vi "CT-Sweep One Component (LUT).vi"(0 "Phase In":dbl=100000.0, 1 "factors":dbl[](array[numeric]), 5 "Last Freq (Hz)":dbl=100000.0, 7 "New Freq (Hz)":dbl=100000.0, 9 "dt (s)":dbl=100000.0, 11 "Npts":i32, 13 "randomize phase":bool) -> (4 "Phase Out":dbl, 8 "Y":dbl[](array[numeric]))   [LabVIEW 2015]
uses:
  CT-Globals.vi
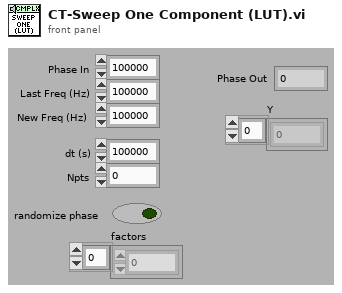
[diagram p1: front panel]
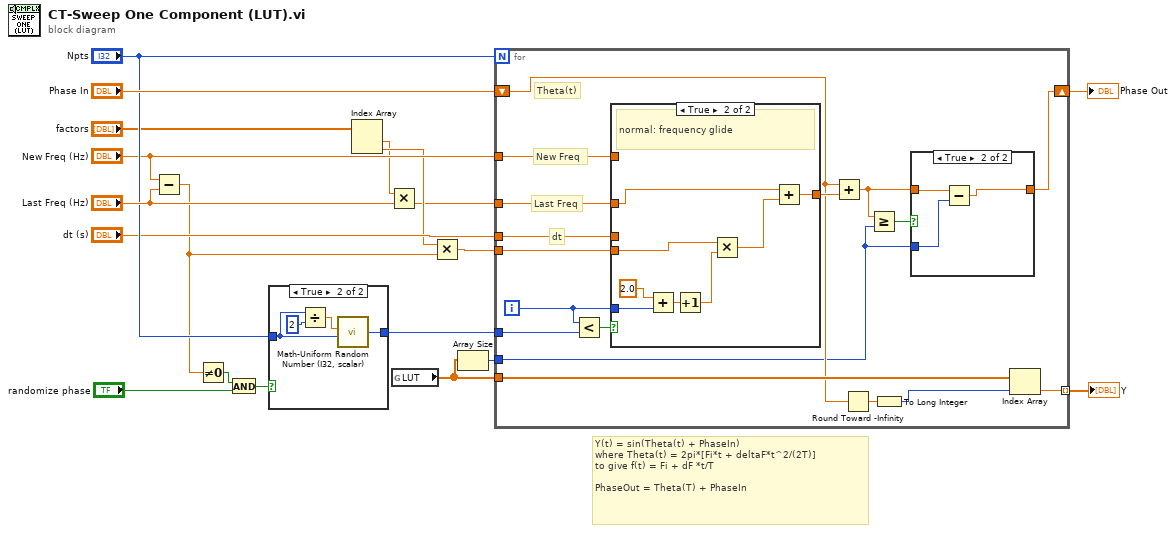
[diagram p0: block diagram]
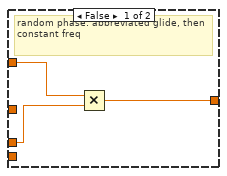
[diagram p4: hidden frame]
diagram:
  # "Y(t) = sin(Theta(t) + PhaseIn)\nwhere Theta(t) = 2pi*[Fi*t + deltaF*t^2/(2T)]\nto give f(t) = Fi + dF *t/T \n\nPhaseOut = Theta(T) + PhaseIn"
  n1 = Subtract(x="New Freq (Hz)", y="Last Freq (Hz)") -> (x-y=w4:dbl)
  n2 = Not Equal To 0?(x=w4) -> (x != 0?=w12:bool)
  n3 = And(x=w12, y="randomize phase") -> (x .and. y?=w13:bool)
  n4 = case shown="True" w13 {
    tunnel: "Npts" -> [w20 w23]
    tunnel: [w20 w21] -> w14
    frame False {
    }
    frame True {
      n5 = Divide(x=w23, y=2) -> (x/y=w22:dbl)
      n6 = call "Math-Uniform Random Number (I32, scalar).vi"("Ymax"=w23, "Ymin"=w22) -> ("Random Int"=w21:i32)  [unwired: 4 in]
    }
  }
  n7 = Index Array(array="factors") -> (element #1=w1:dbl, element #2=w5:dbl)  [unwired: 2 in]
  n8 = Multiply(x=w1, y="Last Freq (Hz)") -> (x*y=w2:dbl)
  n9 = global read "CT-Globals.vi" "LUT"() -> (w8:dbl[])
  n10 = Multiply(x=w5, y=w4) -> (x*y=w3:dbl)
  n11 = Array Size(array=w8) -> (size(s)=w9:i32)
  n12 = for {
    N: "Npts" -> [_]
    tunnel: "dt (s)" -> [w40]
    shift-right: [w26] -> w17
    shift-left: "Phase In" -> [w32]
    tunnel: w2 -> [w41]
    tunnel: [w33] -> w10 mode=indexing
    tunnel: w14 -> [w37]
    tunnel: "New Freq (Hz)" -> [w36]
    tunnel: w8 -> [w34]
    tunnel: w9 -> [w25]
    tunnel: w3 -> [w29]
    i -> [w38]
    # "New Freq"
    # "dt"
    # "Theta(t)"
    # "Last Freq"
    n13 = Less?(x=w38, y=w37) -> (x < y?=w35:bool)
    n14 = case shown="True" w35 {
      tunnel: w41 -> [_ w56]
      tunnel: w40 -> [w48 _]
      tunnel: [w47 w55] -> w39
      tunnel: w38 -> [_ w54]
      tunnel: w36 -> [w46 _]
      tunnel: w29 -> [_ w50]
      frame False {
        # "random phase: abbreviated glide, then constant freq"
        n15 = Multiply(x=w46, y=w48) -> (x*y=w47:dbl)
      }
      frame True {
        # "normal: frequency glide"
        n16 = Add(x=2.0, y=w54) -> (x+y=w52:dbl)
        n17 = Increment(x=w52) -> (x+1=w51:dbl)
        n18 = Multiply(x=w50, y=w51) -> (x*y=w49:dbl)
        n19 = Add(x=w56, y=w49) -> (x+y=w55:dbl)
      }
    }
    n20 = Add(x=w32, y=w39) -> (x+y=w27:dbl)
    n21 = Round Toward -Infinity(1:w32) -> (0:w30:dbl)
    n22 = Greater Or Equal?(x=w27, y=w25) -> (x >= y?=w28:bool)
    n23 = To Long Integer(number=w30) -> (32bit integer=w31:i32)
    n24 = case shown="True" w28 {
      tunnel: w27 -> [w42 w45]
      tunnel: [w42 w43] -> w26
      tunnel: w25 -> [_ w44]
      frame False {
      }
      frame True {
        n25 = Subtract(x=w45, y=w44) -> (x-y=w43:dbl)
      }
    }
    n26 = Index Array(array=w34, index=w31) -> (element=w33:dbl)
  }
  "Y" <- w10
  "Phase Out" <- w17
